vi "fronts64.vi"(3 "IN":u64 format="%x") -> (0 "FALL":u64 format="%x", 1 "RAISE":u64 format="%x")   [LabVIEW 2019, in "Logik.lvlib"]
uses:
  Logik.lvlib
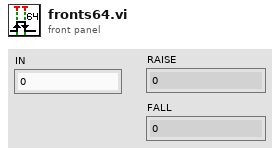
[diagram p1: front panel]
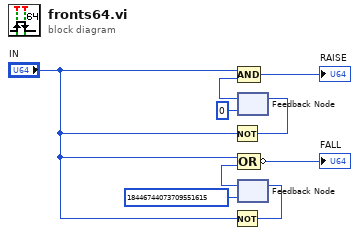
[diagram p0: block diagram]
diagram:
  n1 = Not(x="IN") -> (.not. x?=w9:u64)
  n2 = Not(x="IN") -> (.not. x?=w7:u64)
  n3 = feedback #1(u64 0) -> (w8:u64)
  n4 = Compound Arithmetic op=AND("IN", w8) -> (→"RAISE":u64)
  n5 = feedback-in #1(w9) -> ()
  n6 = feedback #2(u64 18446744073709551615) -> (w6:u64)
  n7 = Compound Arithmetic op=OR("IN", w6) -> (invert →"FALL":u64)
  n8 = feedback-in #2(w7) -> ()
